vi "capture_single_color_dual_view (SubVI).vi"(0 "SpimA path":path, 1 "Control values":T4, 2 "volume number":i32, 3 "filename prefix":string, 4 "Cam A handle in":u32, 5 "Capture on/off":bool, 6 "Cam A error in":errorcluster, 7 "Cam B error in":errorcluster, 8 "SpimB path":path, 9 "Stage 1 time cluster":T2, 10 "Cam B handle in":u32, 11 "Stage 1 DAQ cluster":T3, 13 "Stage 2 time cluster":T1, 15 "stage 2 DAQ cluster":T3) -> (12 "Stage 0":u32, 14 "Stage 1":u32, 16 "Stage 2":u32, 18 "Stage 3":u32, 19 "Cam B Frame Count":i32, 20 "Camera A error out":errorcluster, 21 "DAC card stage A error":errorcluster, 22 "DAC card stage B error":errorcluster, 23 "interstage":u32, 24 "Camera A handle":u32, 25 "Camera B handle":u32, 26 "Cam A Frame Count":i32, 27 "Camera B error out":errorcluster)   [LabVIEW 2016]
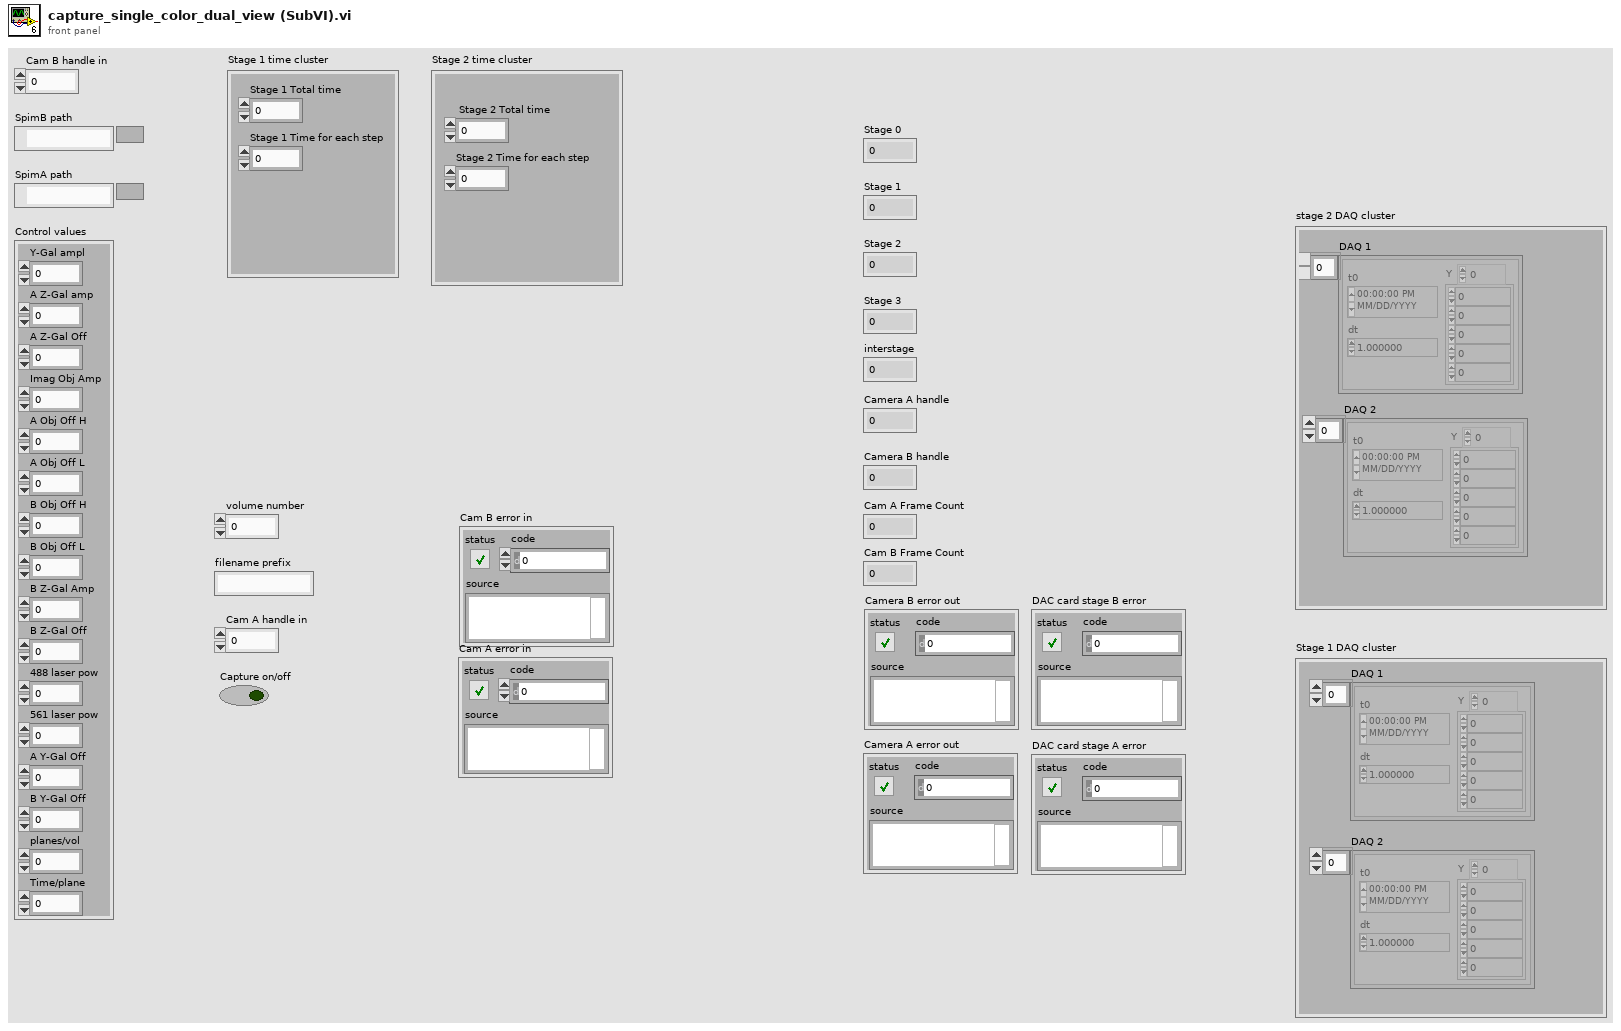
[diagram p1: front panel]
types:
  T1 = cluster{" Stage 2 Total time":dbl, "Stage 2 Time for each step":dbl}
  T2 = cluster{"Stage 1 Total time":dbl, "Stage 1 Time for each step":dbl}
  T3 = cluster{"DAQ 1":waveform(dbl)[], "DAQ 2":waveform(dbl)[]}
  T4 = cluster{"Y-Gal ampl":dbl, "A Z-Gal amp":dbl, "A Z-Gal Off":dbl, "Imag Obj Amp":dbl, "A Obj Off H":dbl, "A Obj Off L":dbl, "B Obj Off H":dbl, "B Obj Off L":dbl, "B Z-Gal Amp":dbl, "B Z-Gal Off":dbl, "488 laser pow":dbl, "561 laser pow":dbl, "A Y-Gal Off":dbl, "B Y-Gal Off ":dbl, "planes/vol":dbl, "Time/plane":dbl}
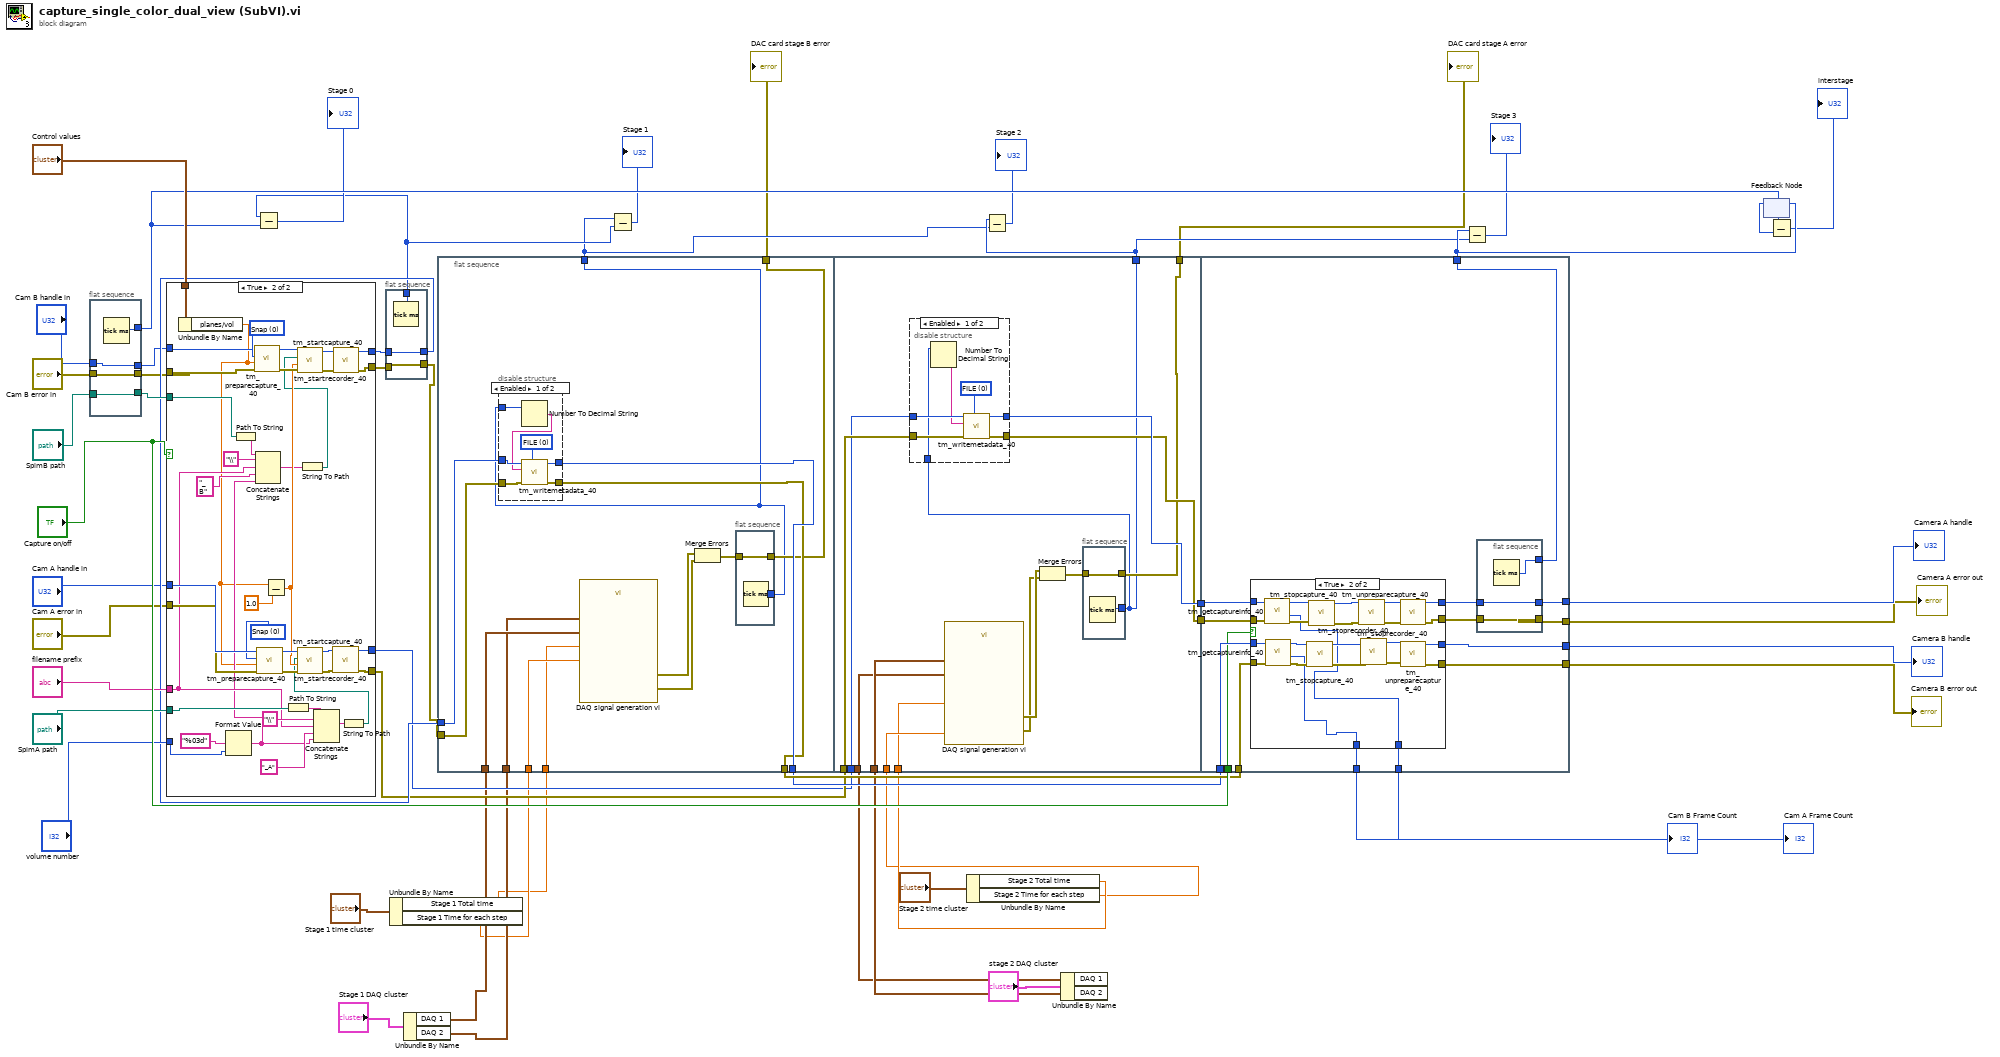
[diagram p0: block diagram]
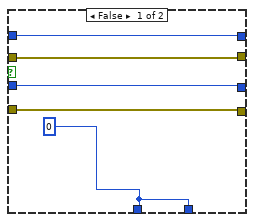
[diagram p5: hidden frame]
diagram:
  n1 = flat-sequence {
    tunnel: [w58] -> w33
    tunnel: "Cam B handle in" -> [w58]
    tunnel: [w57] -> w35
    tunnel: "Cam B error in" -> [w57]
    tunnel: [w56] -> w40
    tunnel: [w55] -> w47
    tunnel: "SpimB path" -> [w55]
    frame #0 {
      n2 = Tick Count (ms)() -> (millisecond timer value=w56:u32)
    }
  }
  n3 = case shown="True" "Capture on/off" {
    tunnel: "Cam A handle in" -> [w60 w94]
    tunnel: "Cam A error in" -> [w59 w93]
    tunnel: [w60 w65] -> w13
    tunnel: [w59 w63] -> w14
    tunnel: [w62 w90] -> w23
    tunnel: [w61 w89] -> w24
    tunnel: w33 -> [w62 w88]
    tunnel: w35 -> [w61 w87]
    tunnel: "SpimA path" -> [_ w79]
    tunnel: "volume number" -> [_ w78]
    tunnel: "filename prefix" -> [_ w71]
    tunnel: w47 -> [_ w69]
    tunnel: "Control values" -> [_ w68]
    frame False {
    }
    frame True {
      w91 = 0 items=["Snap", "Sequence"] ("Capture mode")
      w92 = 0 items=["Snap", "Sequence"] ("Capture mode")
      n4 = Unbundle By Name(w68) -> ("planes/vol"=w67:dbl)
      n5 = Format Value(format string="%03d", value (0)=w78) -> (output string=w70:string)  [unwired: 1 in]
      n6 = Path To String(path=w69) -> (string=w75:string)
      n7 = call <userlib>:"tm_preparecapture_40.vi"("error in (no error)"=w87, "Frames"=w67, "Capture mode"=w92, "Handle in"=w88) -> ("error out"=w98:errorcluster, "Handle out"=w97:u32)  [unwired: 4 in, 2 out]
      n8 = Concatenate Strings(w75, "\\", w71, "_B" ("string"), w70) -> (w74:string)
      n9 = call <userlib>:"tm_preparecapture_40.vi"("error in (no error)"=w93, "Frames"=w67, "Capture mode"=w91, "Handle in"=w94) -> ("error out"=w96:errorcluster, "Handle out"=w95:u32)  [unwired: 4 in, 2 out]
      n10 = Subtract(x=w67, y=1.0) -> (x-y=w85:dbl)
      n11 = Path To String(path=w79) -> (string=w83:string)
      n12 = String To Path(string=w74) -> (path=w72:path)
      n13 = call <userlib>:"tm_startrecorder_40.vi"("error in (no error)"=w98, "frames"=w85, "File"=w72, "Handle in"=w97) -> ("error out"=w100:errorcluster, "Handle out"=w99:u32)  [unwired: 6 in]
      n14 = Concatenate Strings(w83, "\\", w71, "_A" ("string"), w70) -> (w84:string)
      n15 = call <userlib>:"tm_startcapture_40.vi"("error in (no error)"=w100, "Handle in"=w99) -> ("error out"=w89:errorcluster, "Handle out"=w90:u32)  [unwired: 8 in]
      n16 = String To Path(string=w84) -> (path=w80:path)
      n17 = call <userlib>:"tm_startrecorder_40.vi"("error in (no error)"=w96, "frames"=w85, "File"=w80, "Handle in"=w95) -> ("error out"=w64:errorcluster, "Handle out"=w66:u32)  [unwired: 6 in]
      n18 = call <userlib>:"tm_startcapture_40.vi"("error in (no error)"=w64, "Handle in"=w66) -> ("error out"=w63:errorcluster, "Handle out"=w65:u32)  [unwired: 8 in]
    }
  }
  n19 = Subtract(x=w37, y=w40) -> (x-y=→"Stage 0":u32)
  n20 = flat-sequence {
    tunnel: [w103] -> w44
    tunnel: w23 -> [w103]
    tunnel: [w102] -> w42
    tunnel: w24 -> [w102]
    tunnel: [w101] -> w37
    frame #0 {
      n21 = Tick Count (ms)() -> (millisecond timer value=w101:u32)
    }
  }
  n22 = Unbundle By Name("Stage 1 time cluster") -> ("Stage 1 Total time"=w5:dbl, "Stage 1 Time for each step"=w4:dbl)
  n23 = Unbundle By Name("Stage 1 DAQ cluster") -> ("DAQ 1"=w7:waveform(dbl)[], "DAQ 2"=w8:waveform(dbl)[])
  n24 = flat-sequence {
    tunnel: [w105] -> w17
    tunnel: [w113] -> w41
    tunnel: [w104] -> w27
    tunnel: w42 -> [w112]
    tunnel: [w111] -> w43
    tunnel: w44 -> [w114]
    tunnel: w5 -> [w110]
    tunnel: w4 -> [w109]
    tunnel: w7 -> [w108]
    tunnel: w8 -> [w107]
    tunnel: [w138] -> w54
    tunnel: [w137] -> w53
    tunnel: [w130] -> w22
    tunnel: [w128] -> w28
    tunnel: w14 -> [w136]
    tunnel: w13 -> [w135]
    tunnel: w1 -> [w134]
    tunnel: w2 -> [w133]
    tunnel: w10 -> [w131]
    tunnel: w11 -> [w132]
    tunnel: w54 -> [w164]
    tunnel: w53 -> [w163]
    tunnel: w43 -> [w165]
    tunnel: [w162] -> w18
    tunnel: [w161] -> w19
    tunnel: [w160] -> w20
    tunnel: [w158] -> w21
    tunnel: [w156] -> w31
    tunnel: w41 -> [w155]
    tunnel: "Capture on/off" -> [w154]
    tunnel: [w153] -> w51
    tunnel: [w152] -> w52
    frame #0 {
      n25 = disable-structure shown="Enabled" {
        disable-tunnel: w114 -> [w125 w127]
        disable-tunnel: [w124 w127] -> w113
        disable-tunnel: w112 -> [w123 w126]
        disable-tunnel: [w122 w126] -> w111
        disable-tunnel: w104 -> [w120 _]
        frame Enabled {
          w121 = 0 items=["FILE"=0, "FRAME"=2] ("Type")
          n26 = Number To Decimal String(number=w120) -> (decimal integer string=w119:string)  [unwired: 1 in]
          n27 = call <userlib>:"tm_writemetadata_40.vi"("Type"=w121, "error in (no error)"=w123, "Metadata"=w119, "Handle"=w125) -> ("error out"=w122:errorcluster, "Handle"=w124:u32)  [unwired: 6 in]
        }
        frame Disabled {
        }
      }
      n28 = call "DAQ signal generation vi.vi"("Time for each step"=w109, "Total time"=w110, "DAQ 1"=w108, "DAQ 2"=w107) -> ("error out"=w116:errorcluster, "error out 7"=w115:errorcluster)  [unwired: 6 in]
      n29 = Merge Errors(w116, w115) -> (w106:errorcluster)
      n30 = flat-sequence {
        tunnel: [w118] -> w105
        tunnel: w106 -> [w118]
        tunnel: [w117] -> w104
        frame #0 {
          n31 = Tick Count (ms)() -> (millisecond timer value=w117:u32)
        }
      }
    }
    frame #1 {
      n32 = disable-structure shown="Enabled" {
        disable-tunnel: [w147 w149] -> w138
        disable-tunnel: [w146 w148] -> w137
        disable-tunnel: w136 -> [w145 w148]
        disable-tunnel: w135 -> [w144 w149]
        disable-tunnel: w128 -> [w141 _]
        frame Enabled {
          w142 = 0 items=["FILE"=0, "FRAME"=2] ("Type")
          n33 = Number To Decimal String(number=w141) -> (decimal integer string=w143:string)  [unwired: 1 in]
          n34 = call <userlib>:"tm_writemetadata_40.vi"("Type"=w142, "error in (no error)"=w145, "Metadata"=w143, "Handle"=w144) -> ("error out"=w146:errorcluster, "Handle"=w147:u32)  [unwired: 6 in]
        }
        frame Disabled {
        }
      }
      n35 = call "DAQ signal generation vi.vi"("Time for each step"=w134, "Total time"=w133, "DAQ 1"=w131, "DAQ 2"=w132) -> ("error out"=w140:errorcluster, "error out 7"=w139:errorcluster)  [unwired: 6 in]
      n36 = Merge Errors(w140, w139) -> (w129:errorcluster)
      n37 = flat-sequence {
        tunnel: [w151] -> w130
        tunnel: w129 -> [w151]
        tunnel: [w150] -> w128
        frame #0 {
          n38 = Tick Count (ms)() -> (millisecond timer value=w150:u32)
        }
      }
    }
    frame #2 {
      n39 = case shown="True" w154 {
        tunnel: w165 -> [w167 w180]
        tunnel: w164 -> [w170 w179]
        tunnel: w163 -> [w169 w178]
        tunnel: [w167 w177] -> w162
        tunnel: [w168 w176] -> w161
        tunnel: [w169 w175] -> w159
        tunnel: [w170 w174] -> w157
        tunnel: w155 -> [w168 w173]
        tunnel: [w166 w172] -> w153
        tunnel: [w166 w171] -> w152
        frame False {
          w166 = 0 ("Frame Count")
        }
        frame True {
          n40 = call <userlib>:"tm_getcaptureinfo_40.vi"("error in (no error)"=w178, "Handle in"=w179) -> ("error out"=w183:errorcluster, "Frame Count"=w171:i32, "Handle out"=w184:u32)  [unwired: 6 in, 1 out]
          n41 = call <userlib>:"tm_getcaptureinfo_40.vi"("error in (no error)"=w180, "Handle in"=w173) -> ("error out"=w181:errorcluster, "Frame Count"=w172:i32, "Handle out"=w182:u32)  [unwired: 6 in, 1 out]
          n42 = call <userlib>:"tm_stopcapture_40.vi"("error in (no error)"=w181, "Handle in"=w182) -> ("error out"=w187:errorcluster, "Handle out"=w188:u32)  [unwired: 8 in]
          n43 = call <userlib>:"tm_stopcapture_40.vi"("error in (no error)"=w183, "Handle in"=w184) -> ("error out"=w191:errorcluster, "Handle out"=w192:u32)  [unwired: 8 in]
          n44 = call <userlib>:"tm_stoprecorder_40.vi"("error in (no error)"=w191, "Handle in"=w192) -> ("error out"=w189:errorcluster, "Handle out"=w190:u32)  [unwired: 8 in]
          n45 = call <userlib>:"tm_stoprecorder_40.vi"("error in (no error)"=w187, "Handle in"=w188) -> ("error out"=w185:errorcluster, "Handle out"=w186:u32)  [unwired: 8 in]
          n46 = call <userlib>:"tm_unpreparecapture_40.vi"("error in (no error)"=w189, "Handle in"=w190) -> ("error out"=w175:errorcluster, "Handle out"=w174:u32)  [unwired: 8 in]
          n47 = call <userlib>:"tm_unpreparecapture_40.vi"("error in (no error)"=w185, "Handle in"=w186) -> ("error out"=w177:errorcluster, "Handle out"=w176:u32)  [unwired: 8 in]
        }
      }
      n48 = flat-sequence {
        tunnel: [w195] -> w160
        tunnel: w159 -> [w195]
        tunnel: [w194] -> w158
        tunnel: w157 -> [w194]
        tunnel: [w193] -> w156
        frame #0 {
          n49 = Tick Count (ms)() -> (millisecond timer value=w193:u32)
        }
      }
    }
  }
  n50 = Subtract(x=w27, y=w37) -> (x-y=→"Stage 1":u32)
  n51 = Unbundle By Name("Stage 2 time cluster") -> ("Stage 2 Total time"=w2:dbl, "Stage 2 Time for each step"=w1:dbl)
  n52 = Subtract(x=w28, y=w27) -> (x-y=→"Stage 2":u32)
  n53 = Unbundle By Name("stage 2 DAQ cluster") -> ("DAQ 1"=w10:waveform(dbl)[], "DAQ 2"=w11:waveform(dbl)[])
  n54 = Subtract(x=w31, y=w28) -> (x-y=→"Stage 3":u32)
  n55 = feedback #1() -> (w32:u32)  [unwired: 1 in]
  n56 = feedback-in #1(w31) -> ()
  n57 = Subtract(x=w40, y=w32) -> (x-y=→"interstage":u32)
  "Cam A Frame Count" <- w52
  "Cam B Frame Count" <- w51
  "DAC card stage A error" <- w22
  "Camera A handle" <- w21
  "Camera A error out" <- w20
  "Camera B handle" <- w19
  "Camera B error out" <- w18
  "DAC card stage B error" <- w17
